vi "Currentvstime.vi"() -> ()   [LabVIEW 2018]
uses:
  <userlib>/KE237.LLB/Keith 237 Operate/Standby.vi
  <vilib>/Utility/file.llb/Write To Spreadsheet File (string).vi
  <instrlib>/Keithley 24XX/Keithley 24XX.lvlib
  <vilib>/Analysis/NI_AALBase.lvlib
panel:
  in  "Measurement Gate Bias (V)":dbl=-0.85 format="%#.3g"
  in  "Initial Gate Bias (V)":dbl format="%#.3g"
  in  "Voltage Compliance Limit 237 (V)":dbl=10.0 format="%#.3f"
  in  "Current Compliance\nLimit 237 (A)":dbl=0.1 format="%#.3f"
  in  "Delay Gate (s)":dbl=60.0 format="%#.3g"
  in  "Autozero? 2":u16(ring) items=["On", "Off", "Once"]
  in  "Measurement Speed (1 PLC) 2":dbl=1.0 format="%.2g"
  in  "Manual Range (Max I) 2":dbl=1.0
  in  "Enable Meas Auto Range 2":bool=TRUE
  in  "Source Mode 2":u16(ring) items=["Voltage", "Current"]
  in  "Keithley 237 GPIB address":string="17"
  in  "Wait Time Btwn Keithley Readings (ms)":i32=30
  out "Time Btwn Iterations (ms)":i32
  out "Total Elapsed Time (ms)":i32
  out "# Avgs":i32
  out "Current (A)":dbl format="%.2e"
  in  "Total Measure Time (s)":dbl=60.0 format="%#.3g"
  in  "Drain Bias (V)":dbl=-0.6 format="%#.3g"
  in  "Current Compliance\nLimit (A)":dbl=0.5 format="%#.3e"
  in  "Keithley 2400\nVISA resource":refnum<visa-resource-name>="GPIB0::24::INSTR"
  in  "Active Area (cm^2)":dbl=0.0122 min=0.0 format="%#.4e"
  in  "ApproximateTime Step (ms)":dbl=300.0 format="%#.3g"
  out "Current Density (mA/cm^2)":dbl format="%.2e"
  in  "Show Current:":enum32{"Density (mA/cm^2)", "Absolute (A)"}(radio)=enum."Absolute (A)"
  in  "Current Offset":dbl format="%^#_3e"
  out "I-t Measurement\nBy M. Ziffer 7/3/2014":cluster{dbl[], dbl[]}(graph)={[-2.0, -1.95, -1.9, -1.85, -1.8, -1.75, -1.7, -1.65, -1.6, -1.55, -1.5, -1.45, -1.4, -1.35, -1.2999999999999998, -1.25, -1.2, -1.15, -1.1, -1.0499999999999998, -1.0, -0.95, -0.8999999999999999, -0.8499999999999999, -0.7999999999999998, -0.75, -0.7, -0.6499999999999999, -0.5999999999999999, -0.5499999999999998, -0.5, -0.44999999999999996, -0.3999999999999999, -0.34999999999999987, -0.2999999999999998, -0.25, -0.19999999999999996, -0.1499999999999999, -0.09999999999999987, -0.04999999999999982, 0.0, 0.050000000000000266, 0.10000000000000009, 0.1499999999999999, 0.20000000000000018, 0.25, 0.30000000000000027, 0.3500000000000001, 0.40000000000000036, 0.4500000000000002, 0.5, 0.5500000000000003, 0.6000000000000001, 0.6500000000000004, 0.7000000000000002, 0.75, 0.8000000000000003, 0.8500000000000001, 0.9000000000000004, 0.9500000000000002, 1.0, 1.0500000000000003, 1.1, 1.1500000000000004, 1.2000000000000002, 1.25, 1.3000000000000003, 1.35, 1.4000000000000004, 1.4500000000000002, 1.5, 1.5500000000000003, 1.6, 1.6500000000000004, 1.7000000000000002, 1.75, 1.8000000000000003, 1.85, 1.9000000000000004, 1.9500000000000002, 2.0, 1.95, 1.9, 1.85, 1.8, 1.75, 1.7, 1.65, 1.6, 1.55, 1.5, 1.45, 1.4, 1.35, 1.2999999999999998, 1.25, 1.2, 1.15, 1.1, 1.0499999999999998, 1.0, 0.95, 0.8999999999999999, 0.8499999999999999, 0.7999999999999998, 0.75, 0.7, 0.6499999999999999, 0.5999999999999999, 0.5499999999999998, 0.5, 0.44999999999999996, 0.3999999999999999, 0.34999999999999987, 0.2999999999999998, 0.25, 0.19999999999999996, 0.1499999999999999, 0.09999999999999987, 0.04999999999999982, 0.0, -0.050000000000000266, -0.10000000000000009, -0.1499999999999999, -0.20000000000000018, -0.25, -0.30000000000000027, -0.3500000000000001, -0.40000000000000036, -0.4500000000000002, -0.5, -0.5500000000000003, -0.6000000000000001, -0.6500000000000004, -0.7000000000000002, -0.75, -0.8000000000000003, -0.8500000000000001, -0.9000000000000004, -0.9500000000000002, -1.0, -1.0500000000000003, -1.1, -1.1500000000000004, -1.2000000000000002, -1.25, -1.3000000000000003, -1.35, -1.4000000000000004, -1.4500000000000002, -1.5, -1.5500000000000003, -1.6, -1.6500000000000004, -1.7000000000000002, -1.75, -1.8000000000000003, -1.85, -1.9000000000000004, -1.9500000000000002, -2.0], [-0.9617289445307117, -0.9618513744908972, -0.9601574911889584, -0.9603488957746004, -0.9598860982876659, -0.9595594700613103, -0.9590290885663679, -0.9586886097902229, -0.9580144940757807, -0.9570474587019399, -0.9571418538143588, -0.9562287187728303, -0.9551771894828052, -0.9535572870291384, -0.9535421571112963, -0.9533114258642045, -0.9520938012261039, -0.9513117179729429, -0.9508812384355169, -0.9504840780921618, -0.9504173840793213, -0.9482281628421478, -0.9464640811713977, -0.9453356785488072, -0.9439408336230415, -0.9428695575652444, -0.9416178906119992, -0.9396031084275935, -0.9378375248899987, -0.9354517815949719, -0.9324159524550173, -0.928767917889437, -0.9245502864168607, -0.9203528467096396, -0.9146985405384399, -0.908595454304189, -0.9012966039381313, -0.8917361646028689, -0.8808115851751085, -0.8684870433493713, -0.853007079283089, -0.8360736418594031, -0.8154860511533626, -0.7920970894092216, -0.7641180332150388, -0.7294003786125389, -0.6854183749419586, -0.6263231964633708, -0.5399961516707377, -0.4044042921440459, -0.19129744134883978, 0.11936942255465804, 0.5420583260977958, 1.0996962734707192, 1.8318907919106253, 2.7834859177196174, 3.9948214605959804, 5.494887344369723, 7.293988211209965, 9.39251059714275, 11.765998658717283, 14.371720946722268, 17.153138293174568, 20.070768287470067, 23.082285540692517, 26.15604905590766, 29.26009131920428, 32.38734131897913, 35.54092126952808, 38.70923397757575, 41.89103456238207, 45.09512285116253, 48.318234786641504, 51.57411300669423, 54.84161623237131, 58.130390342544004, 61.4596508891188, 64.79419021952893, 68.17503711098149, 71.57587551887687, 75.0023346626475, 71.8977923333163, 68.72637799211101, 65.51757272894447, 62.2950059155054, 59.076872390492845, 55.84672949319313, 52.615591470047114, 49.383497814590335, 46.15858586388574, 42.93308596012382, 39.714879010509975, 36.494540522470736, 33.276879251143754, 30.087779593472593, 26.903443634933772, 23.758388169345494, 20.669969771208738, 17.671195580039395, 14.804861569698371, 12.12778391916459, 9.68736655227705, 7.528128139792144, 5.673530623057721, 4.128839936603901, 2.8787577310032053, 1.895544581260216, 1.1383875896205915, 0.5622048852612092, 0.12746496878202787, -0.18928305409978952, -0.4042961076690051, -0.5411369085387429, -0.6286316214282486, -0.6871327837574404, -0.7298882072135505, -0.7640718647157413, -0.7921132761963248, -0.8155779431543743, -0.8358809022810104, -0.8523300154596555, -0.8668520109778625, -0.8802307520791266, -0.8907705198464766, -0.8998007445608903, -0.9078572589377096, -0.9150023626386364, -0.9215738644543149, -0.925261336930741, -0.9288795566582202, -0.9332418679701618, -0.9352489739462505, -0.9376688708058178, -0.9394550911063516, -0.9405290371496502, -0.9430050037047499, -0.9440335043698243, -0.9453382929096107, -0.9473152502994113, -0.9474565926568992, -0.9494901203645137, -0.94896546821346, -0.9503187058651598, -0.9511280452203158, -0.9523093469306558, -0.9532668704811476, -0.9541692143312739, -0.9545545822386634, -0.955485183435348, -0.9561708134622656, -0.956805602515258, -0.9577699122788996, -0.9578049002139094, -0.9580356870856992, -0.958780001168953, -0.9592832934359943, -0.9588639388381576, -0.959203916992021, -0.9603773199952523, -0.9611007191920772, -0.9623172869609168]}
  in  "First bias settle (ms)":dbl=2000.0 format="%#.2f"
  out "Outputfile":path
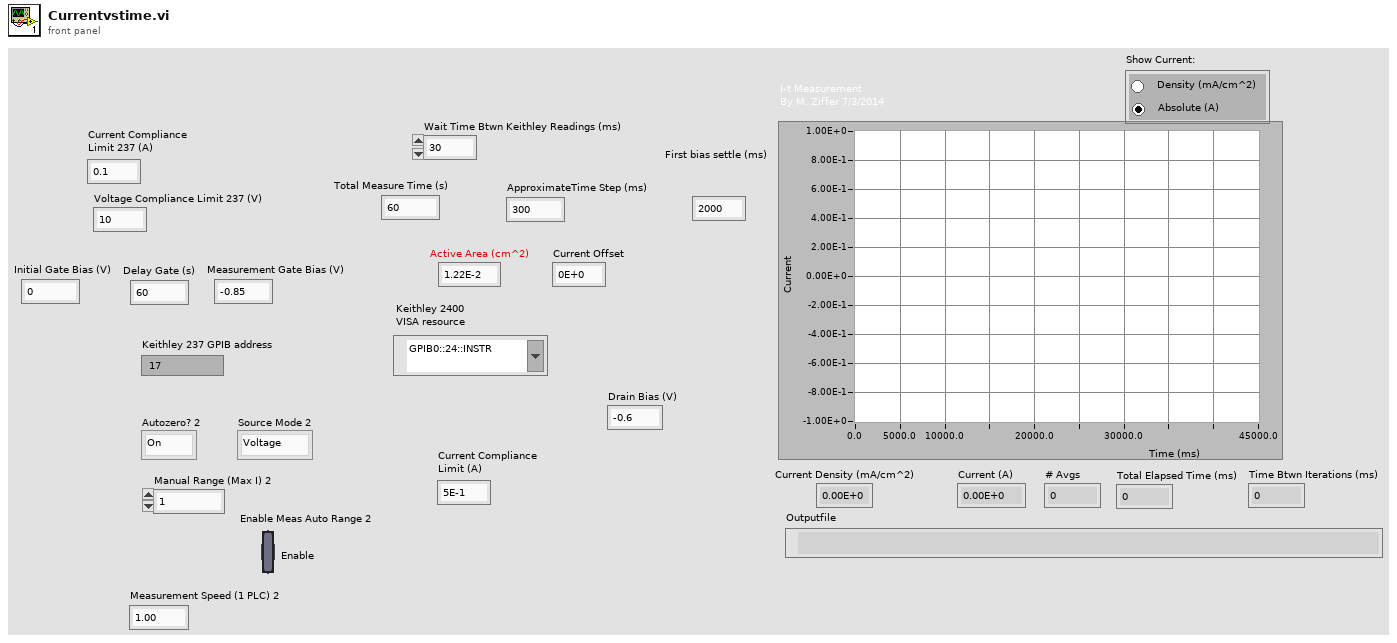
[diagram p1: front panel]
types:
  T1 = cluster{"error":bool, "code":i32, "source":string}
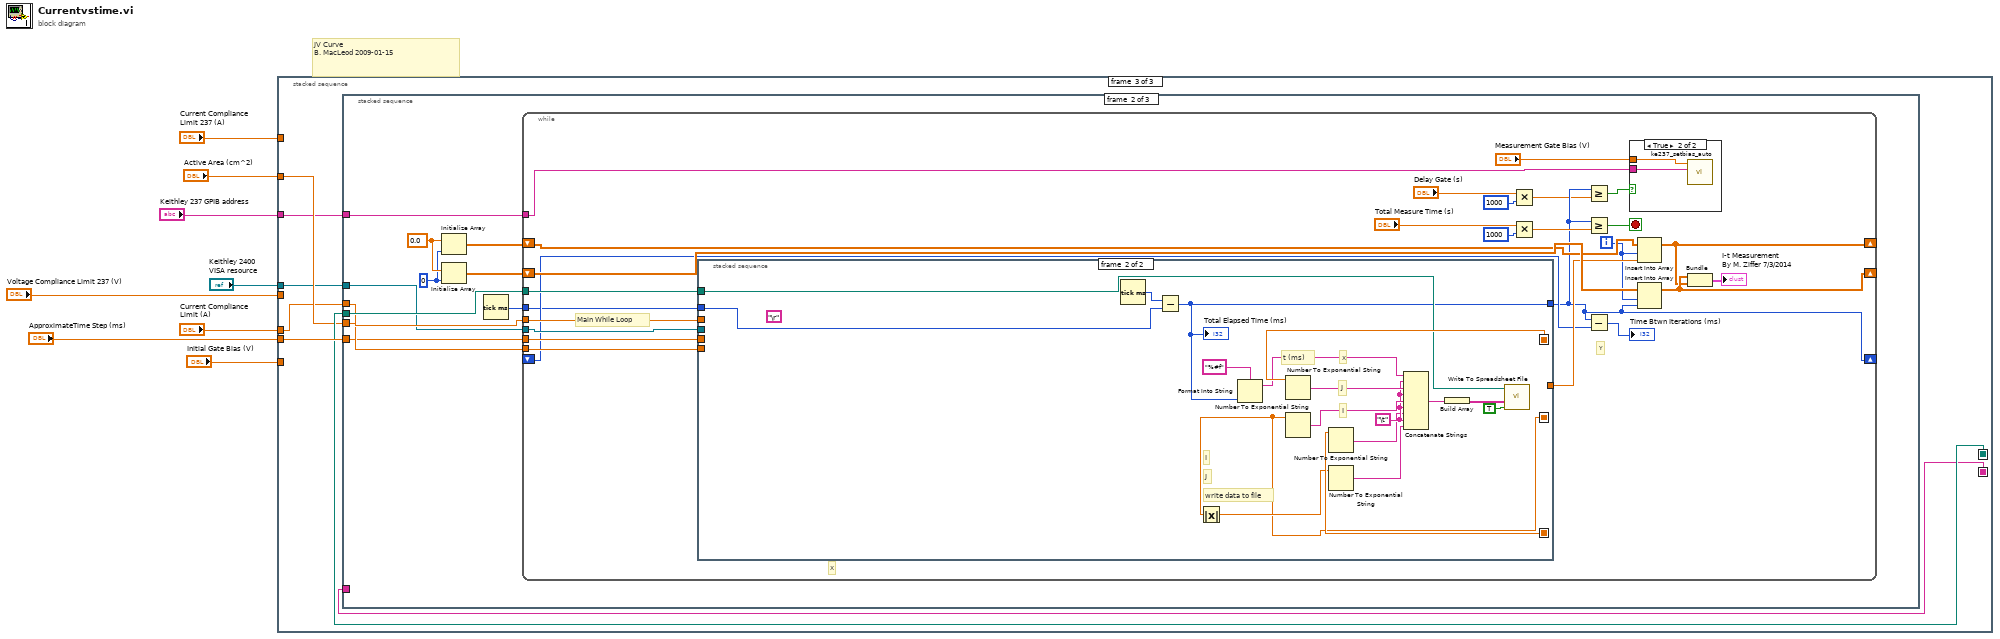
[diagram p0: block diagram]
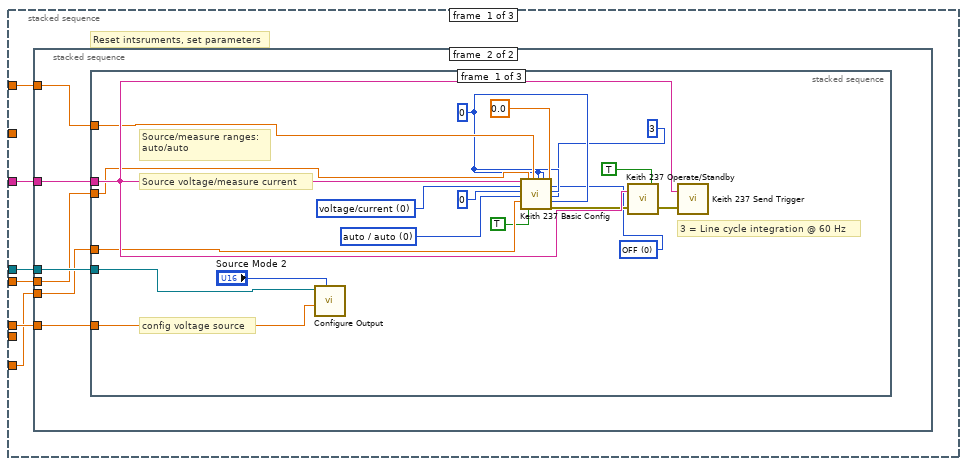
[diagram p2: hidden frame]
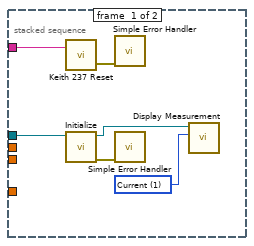
[diagram p3: hidden frame]
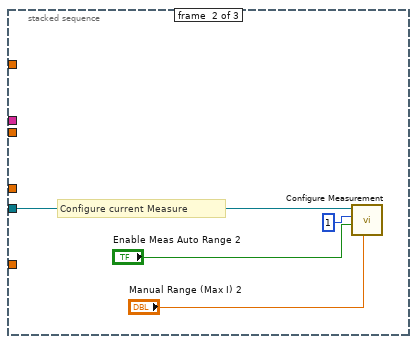
[diagram p4: hidden frame]
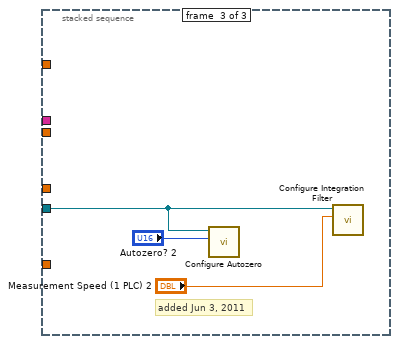
[diagram p5: hidden frame]
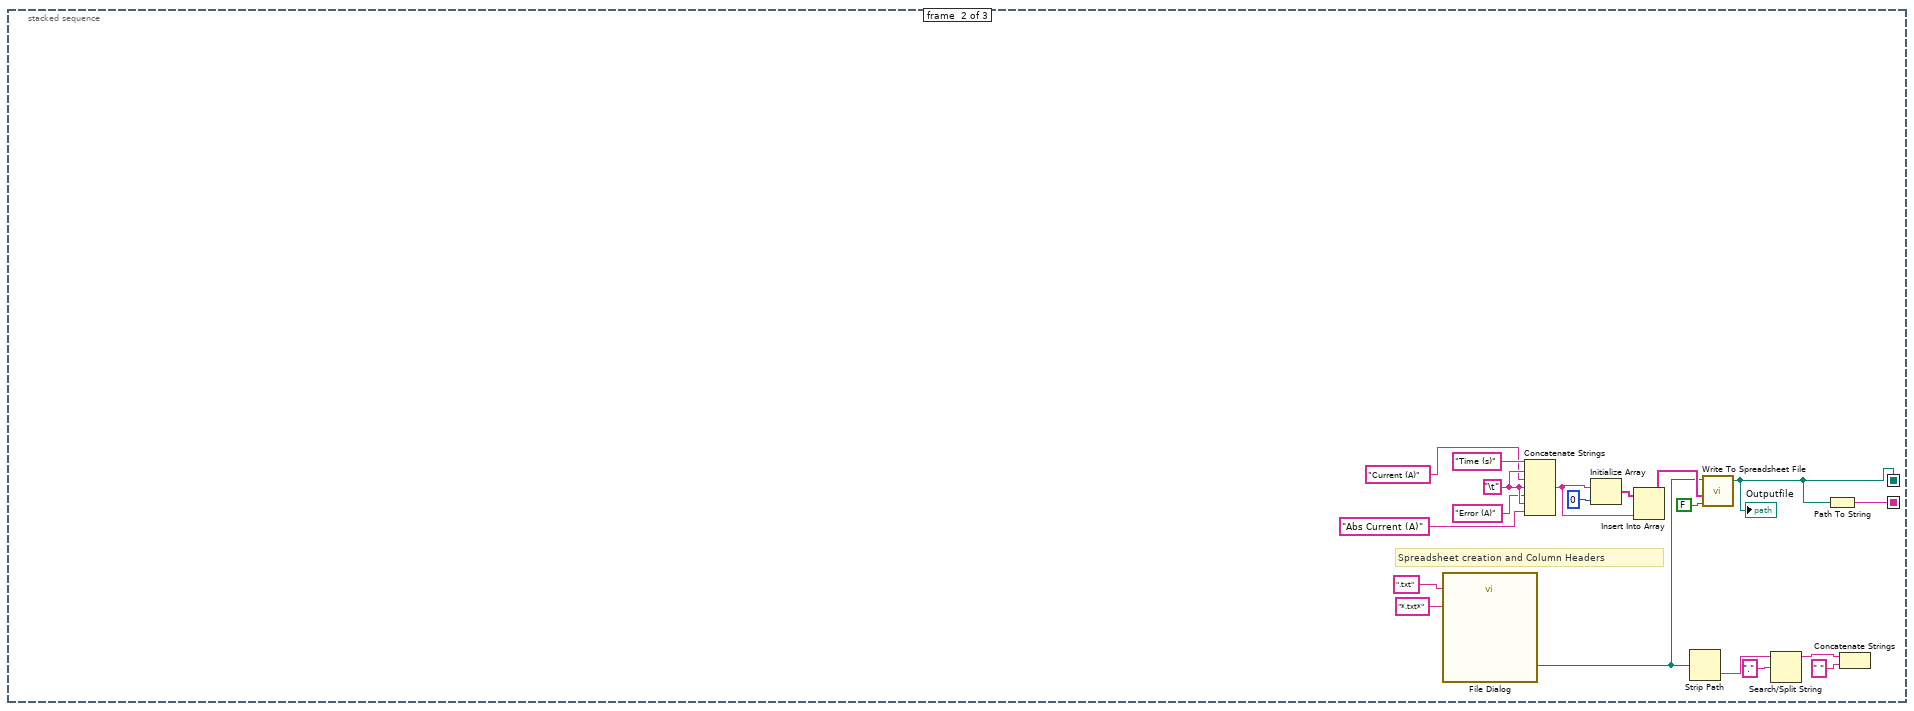
[diagram p6: hidden frame]
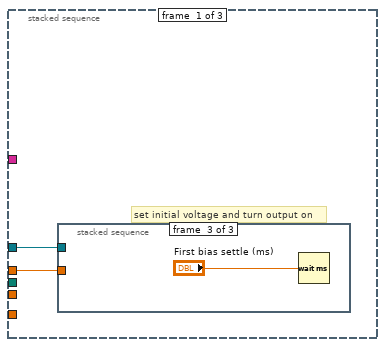
[diagram p7: hidden frame]
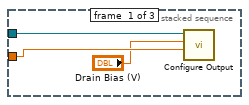
[diagram p8: hidden frame]
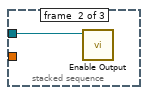
[diagram p9: hidden frame]
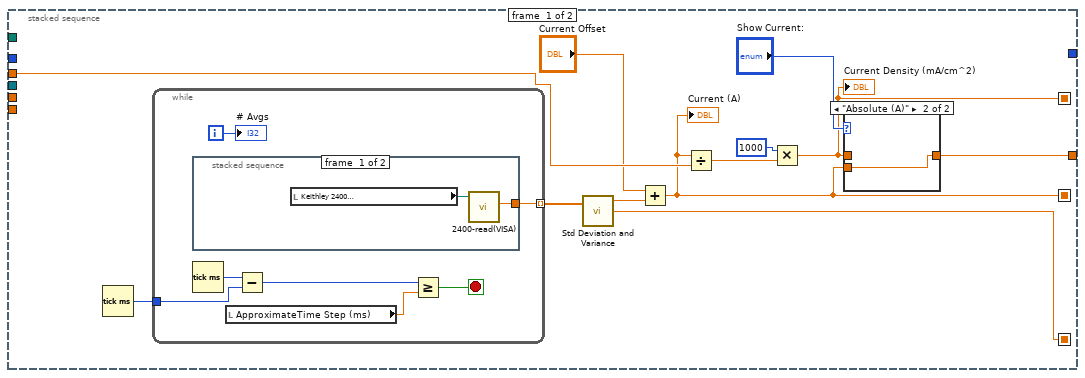
[diagram p11: hidden frame]
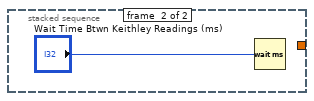
[diagram p12: hidden frame]
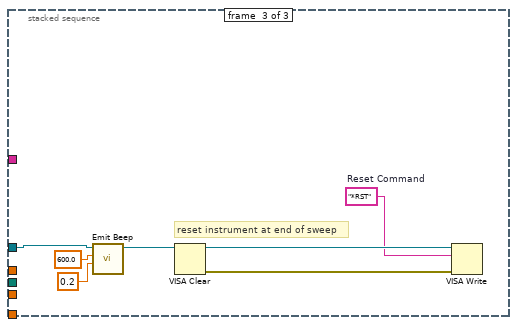
[diagram p14: hidden frame]
diagram:
  # "JV Curve\nB. MacLeod 2009-01-15"
  n1 = stacked-sequence {
    seq-local: [_ w69 _] -> [_ _ w76]
    seq-local: [_ w68 _] -> [_ _ w75]
    tunnel: "ApproximateTime Step (ms)" -> [_ _ w77]
    tunnel: "Active Area (cm^2)" -> [_ _ w74]
    tunnel: "Keithley 2400\nVISA resource" -> [w13 _ w72]
    tunnel: "Current Compliance\nLimit (A)" -> [w14 _ w73]
    tunnel: "Keithley 237 GPIB address" -> [w12 _ w71]
    tunnel: "Voltage Compliance Limit 237 (V)" -> [w11 _ _]
    tunnel: "Current Compliance\nLimit 237 (A)" -> [w10 _ _]
    tunnel: "Initial Gate Bias (V)" -> [w9 _ _]
    frame #0 {
      # "Reset intsruments, set parameters"
      n2 = stacked-sequence {
        tunnel: w12 -> [w19 w24]
        tunnel: w13 -> [w18 w26]
        tunnel: w14 -> [_ w25]
        tunnel: w11 -> [_ w23]
        tunnel: w10 -> [_ w22]
        tunnel: w9 -> [_ w21]
        frame #0 {
          w17 = u16 1 items=["Voltage", "Current", "Resistance"] ("Displayed Measurement (0: Voltage)")
          n3 = call <userlib>:"Keith 237 Reset.vi"("GPIB address"=w19) -> ("error out"=w20:T1)  [unwired: 1 in]
          n4 = call <instrlib>:"Initialize.vi"("VISA resource name"=w18) -> ("error out"=w15:errorcluster, "VISA resource name out"=w16:refnum<visa-resource-name>)  [unwired: 9 in]
          n5 = call <vilib>:"Simple Error Handler.vi"("error in (no error)"=w20) -> ()  [unwired: 1 in, 8 out]
          n6 = call <vilib>:"Simple Error Handler.vi"("error in (no error)"=w15) -> ()  [unwired: 1 in, 8 out]
          n7 = call <instrlib>:"Display Measurement.vi"("Displayed Measurement (0: Voltage)"=w17, "VISA resource name"=w16) -> ()  [unwired: 8 in, 2 out]
        }
        frame #1 {
          n8 = stacked-sequence {
            tunnel: w26 -> [w43 w45 w49]
            tunnel: w25 -> [w42 _ _]
            tunnel: w24 -> [w41 _ _]
            tunnel: w23 -> [w40 _ _]
            tunnel: w22 -> [w39 _ _]
            tunnel: w21 -> [w38 _ _]
            frame #0 {
              w28 = u16 0 items=["OFF", "ON"] ("default delay (on:1)")
              w29 = u16 0 items=["auto / auto", "1 nA / 1.1 V", "10 nA / 11 V", "100 nA / 110 V", "0.001 mA / 1100 V", "0.01 mA / 1100 V", "0.1 mA / 1100 V", "1 mA / 1100 V", "10 mA / 1100 V", "100 mA / 1100 V"] ("source range\nI source / V source (auto:0)")
              w30 = u16 0 items=["voltage/current", "current/voltage"] ("source/measure (V/I:0)")
              w32 = u16 0
              # "3 = Line cycle integration @ 60 Hz"
              # "Source/measure ranges:\nauto/auto"
              # "Source voltage/measure current"
              # "config voltage source"
              n9 = call <instrlib>:"Configure Output.vi"("Source Mode  (0: Voltage)"="Source Mode 2", "Compliance  Level (0.1)"=w42, "VISA resource name"=w43) -> ()  [unwired: 3 in, 6 out]
              n10 = call <userlib>:"Keith 237 Basic Config.vi"("GPIB address"=w41, "source/measure (V/I:0)"=w30, "function (DC:0)"=u16 0, "source range\nI source / V source (auto:0)"=w29, "source level"=w38, "voltage \ncompliance level"=w40, "1100 V range (disabled:F)"=TRUE, "current \ncompliance level"=w39, "compliance/\nmeasurement range (auto:0)"=w32, "suppression (off:0)"=w32, "DC delay (sec)"=0.0, "default delay (on:1)"=w28, "filter (disabled:0)"=w32, "integration time (medium:1)"=u16 3, "sense (local:0)"=w32) -> ("error out"=w37:T1)  [unwired: 4 in]
              n11 = call "Keith 237 Operate/Standby.vi"("source"=TRUE, "error in"=w37, "GPIB address"=w41) -> ("error out"=w35:T1)
              n12 = call <userlib>:"Keith 237 Send Trigger.vi"("GPIB address"=w41, "error in"=w35) -> ()  [unwired: 1 out]
            }
            frame #1 {
              # "Configure current Measure"
              n13 = call <instrlib>:"Configure Measurement.vi"("Manual Range (1.0)"="Manual Range (Max I) 2", "Enable Auto Range (T:Enable)"="Enable Meas Auto Range 2", "Function (0: Volts)"=1, "VISA resource name"=w45) -> ()  [unwired: 1 in, 7 out]
            }
            frame #2 {
              # "added Jun 3, 2011"
              n14 = call <instrlib>:"Configure Autozero.vi"("Autozero  (0: On)"="Autozero? 2", "VISA resource name"=w49) -> ()  [unwired: 1 in, 9 out]
              n15 = call <instrlib>:"Configure Integration Filter.vi"("Measurement Speed (1 PLC)"="Measurement Speed (1 PLC) 2", "VISA resource name"=w49) -> ()  [unwired: 8 in, 2 out]
            }
          }
        }
      }
    }
    frame #1 {
      w60 = "\t"
      # "Spreadsheet creation and Column Headers"
      n16 = call "File Dialog"("default name"=".txt", "pattern (all files)"="*.txt*") -> ("selected path"=w57:path)  [unwired: 5 in, 8 out]
      n17 = Concatenate Strings("Time (s)", w60, "Current (A)", w60, "Error (A)", w60, "Abs Current (A)" ("string")) -> (w65:string)
      n18 = Initialize Array(w65, 0 ("dimension size")) -> (w64:string[])
      n19 = Insert Into Array(array=w64, new element=w65) -> (w67:string[])  [unwired: 1 in]
      n20 = Strip Path(path=w57) -> (name=w56:string)  [unwired: 1 out]
      n21 = call-poly <vilib>:"Write To Spreadsheet File.vi"("append to file? (new file:F)"=FALSE, "1D data"=w67, "file path (dialog if empty)"=w57) -> ("new file path (Not A Path if cancelled)"=w69:path)  [unwired: 3 in, 2 out]
      "Outputfile" <- w69
      n22 = Search/Split String(string=w56, search string/char (-)=".") -> (substring before match=w59:string)  [unwired: 3 out]
      n23 = Path To String(path=w69) -> (string=w68:string)
      n24 = Concatenate Strings(w59, " " ("string")) -> ()  [unwired: 1 out]
    }
    frame #2 {
      n25 = stacked-sequence {
        tunnel: w77 -> [_ w87 _]
        tunnel: w76 -> [_ w95 _]
        tunnel: w75 -> [_ _ _]
        tunnel: w74 -> [_ w90 _]
        tunnel: w73 -> [w79 w88 _]
        tunnel: w72 -> [w78 w89 w169]
        tunnel: w71 -> [_ w85 _]
        frame #0 {
          # "set initial voltage and turn output on"
          n26 = stacked-sequence {
            tunnel: w78 -> [w81 w83 _]
            tunnel: w79 -> [w82 _ _]
            frame #0 {
              n27 = call <instrlib>:"Configure Output.vi"("Compliance  Level (0.1)"=w82, "Output Level (0)"="Drain Bias (V)", "VISA resource name"=w81) -> ()  [unwired: 3 in, 6 out]
            }
            frame #1 {
              n28 = call <instrlib>:"Enable Output.vi"("VISA resource name"=w83) -> ()  [unwired: 2 in, 9 out]
            }
            frame #2 {
              n29 = Wait (ms)(milliseconds to wait="First bias settle (ms)") -> ()  [unwired: 1 out]
            }
          }
        }
        frame #1 {
          w91 = 0
          w92 = 0.0
          n30 = Initialize Array(w92, w91) -> (w93:dbl[])
          n31 = Initialize Array(w92, w91) -> (w94:dbl[])
          n32 = Tick Count (ms)() -> (millisecond timer value=w86:u32)
          n33 = while {
            shift-left: w93 -> [w118]
            shift-right: [w112] -> _
            shift-left: w94 -> [w119]
            shift-right: [w114] -> _
            tunnel: w95 -> [w120]
            tunnel: w90 -> [w117]
            tunnel: w89 -> [w116]
            tunnel: w88 -> [w115]
            tunnel: w87 -> [w110]
            tunnel: w86 -> [w103]
            shift-right: [w102] -> _
            shift-left: _ -> [w108]
            tunnel: w85 -> [w96]
            i -> [w111]
            stop <- w109 stop-if-true
            # "Main While Loop"
            # "X"
            # "Y"
            n34 = stacked-sequence {
              seq-local: [w129 _] -> [_ w164]
              seq-local: [w134 _] -> [_ w154]
              seq-local: [w125 _] -> [_ w152]
              tunnel: [w130 _] -> w113
              tunnel: w120 -> [_ w159]
              tunnel: w117 -> [w128 _]
              tunnel: w116 -> [_ _]
              tunnel: w115 -> [_ _]
              tunnel: w110 -> [_ _]
              tunnel: w103 -> [_ w149]
              tunnel: [_ w148] -> w102
              frame #0 {
                n35 = Tick Count (ms)() -> (millisecond timer value=w124:u32)
                n36 = while {
                  tunnel: [w142] -> w135 mode=indexing
                  tunnel: w124 -> [w140]
                  i -> [w141]
                  stop <- w138 stop-if-true
                  n37 = stacked-sequence {
                    tunnel: [w143 _] -> w142
                    frame #0 {
                      n38 = local read "Keithley 2400\nVISA resource"() -> (w144:refnum<visa-resource-name>)
                      n39 = call "2400-read(VISA).vi"("2400 VISA ID"=w144) -> ("Current"=w143:dbl)  [unwired: 6 out]
                    }
                    frame #1 {
                      n40 = Wait (ms)(milliseconds to wait="Wait Time Btwn Keithley Readings (ms)") -> ()  [unwired: 1 out]
                    }
                  }
                  n41 = Tick Count (ms)() -> (millisecond timer value=w137:u32)
                  n42 = local read "ApproximateTime Step (ms)"() -> (w136:dbl)
                  n43 = Subtract(x=w137, y=w140) -> (x-y=w139:u32)
                  n44 = Greater Or Equal?(x=w139, y=w136) -> (x >= y?=w138:bool)
                  "# Avgs" <- w141
                }
                n45 = call <vilib>:"Std Deviation and Variance.vi"("X"=w135) -> ("mean"=w127:dbl, "standard deviation"=w134:dbl)  [unwired: 1 in, 1 out]
                n46 = Add(x="Current Offset", y=w127) -> (x+y=w125:dbl)
                "Current (A)" <- w125
                n47 = Divide(x=w125, y=w128) -> (x/y=w133:dbl)
                n48 = Multiply(x=1000, y=w133) -> (x*y=w129:dbl)
                "Current Density (mA/cm^2)" <- w129
                n49 = case shown="\"Absolute (A)\"" "Show Current:" {
                  tunnel: [w146 w147] -> w130
                  tunnel: w129 -> [w146 _]
                  tunnel: w125 -> [_ w147]
                  frame "Density (mA/cm^2)", Default {
                  }
                  frame "Absolute (A)" {
                  }
                }
              }
              frame #1 {
                (unwired) "\r"
                w156 = "\t"
                # "I"
                # "I"
                # "J"
                # "t (ms)"
                # "J"
                # "write data to file"
                # "X"
                n50 = Tick Count (ms)() -> (millisecond timer value=w150:u32)
                n51 = Subtract(x=w150, y=w149) -> (x-y=w148:u32)
                "Total Elapsed Time (ms)" <- w148
                n52 = Absolute Value(x=w152) -> (abs(x)=w153:dbl)
                n53 = Format Into String(format string="%#f", w148) -> (resulting string=w162:string)  [unwired: 2 in, 1 out]
                n54 = Number To Exponential String(number=w164) -> (E-format string=w165:string)  [unwired: 3 out]
                n55 = Number To Exponential String(number=w152) -> (E-format string=w161:string)  [unwired: 3 out]
                n56 = Number To Exponential String(number=w154) -> (E-format string=w155:string)  [unwired: 3 out]
                n57 = Number To Exponential String(number=w153) -> (E-format string=w151:string)  [unwired: 3 out]
                n58 = Concatenate Strings(w162, w156, w165, w156, w161, w156, w155, w156, w151) -> (w160:string)
                n59 = Build Array(w160) -> (w158:string[])
                n60 = call-poly <vilib>:"Write To Spreadsheet File.vi"("append to file? (new file:F)"=TRUE, "1D data"=w158, "file path (dialog if empty)"=w159) -> ()  [unwired: 3 in, 3 out]
              }
            }
            n61 = Multiply(x="Delay Gate (s)", y=1000) -> (x*y=w101:dbl)
            n62 = Multiply(x="Total Measure Time (s)", y=1000) -> (x*y=w104:dbl)
            n63 = Greater Or Equal?(x=w102, y=w101) -> (x >= y?=w98:bool)
            n64 = Greater Or Equal?(x=w102, y=w104) -> (x >= y?=w109:bool)
            n65 = Subtract(x=w102, y=w108) -> (x-y=→"Time Btwn Iterations (ms)":u32)
            n66 = case shown="True" w98 {
              tunnel: "Measurement Gate Bias (V)" -> [_ w123]
              tunnel: w96 -> [_ w122]
              frame False {
              }
              frame True {
                n67 = call "ke237_setbias_auto.vi"("GPIB address"=w122, "source level"=w123) -> ()  [unwired: 10 in]
              }
            }
            n68 = Insert Into Array(array=w118, index=w111, new element=w113) -> (w112:dbl[])
            n69 = Insert Into Array(array=w119, index=w111, new element=w102) -> (w114:dbl[])
            n70 = Bundle(w114, w112) -> (→"I-t Measurement\nBy M. Ziffer 7/3/2014":cluster{dbl[], dbl[]})  [unwired: 1 out]
          }
        }
        frame #2 {
          w171 = "*RST"  # Reset Command
          # "reset instrument at end of sweep"
          n71 = call <instrlib>:"Emit Beep.vi"("Beep Duration (.25 s)"=0.2, "Beep Frequency (300)"=600.0, "VISA resource name"=w169) -> ("VISA resource name out"=w168:refnum<visa-resource-name>)  [unwired: 7 in, 1 out]
          n72 = VISA Clear(VISA resource name=w168) -> (VISA resource name out=w172:refnum<visa-resource-name>, error out=w170:errorcluster)  [unwired: 1 in]
          n73 = VISA Write(VISA resource name=w172, write buffer=w171, error in (no error)=w170) -> ()  [unwired: 3 out]
        }
      }
    }
  }
